vi "Test connection.vi"() -> ()   [LabVIEW 2016]
doc: "This example open a connection to the Nanonis Control Software and get the current \"Session path\".\n\n- Nanonis Programming Interface -"
uses:
  Nanonis Prog Interface.lvlib
panel:
  out "Connection status":bool
  in  "Machine name (localhost)":string="localhost"
  out "Session path":path
  # "Example program for the Nanonis SPM Control software programming interface\n(see diagram)."
  # "Connect to the Nanonis Control Software and get the current \"Session path\""
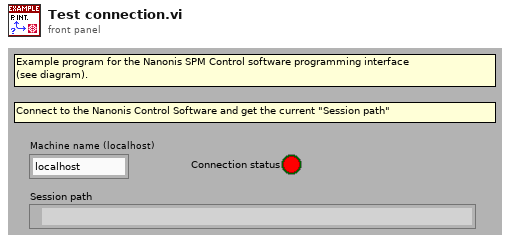
[diagram p1: front panel]
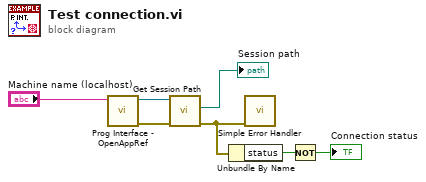
[diagram p0: block diagram]
diagram:
  n1 = call <userlib>:"Prog Interface - OpenAppRef.vi"("Machine name (local machine IP)"="Machine name (localhost)") -> ("Error out"=w6:errorcluster, "Application reference"=w1:refnum<vi>)  [unwired: 5 in]
  n2 = call <userlib>:"Get Session Path.vi"("error in (no error)"=w6, "Application ref in"=w1) -> ("error out"=w4:errorcluster, "Session path"=→"Session path":path)  [unwired: 7 in, 1 out]
  n3 = Unbundle By Name(w4) -> ("status"=w3:bool)
  n4 = call <vilib>:"Simple Error Handler.vi"("error in (no error)"=w4) -> ()  [unwired: 4 in, 5 out]
  n5 = Not(x=w3) -> (.not. x?=→"Connection status":bool)
